vi "Read Attribute Data.vi"(8 "error in (no error)":errorcluster, 10 "Object Name":string, 11 "BNT_BlowfishFactory in":refnum<class "BNT_BlowfishFactory.lvclass">) -> (0 "error out":errorcluster, 2 "Attribute Data":variant, 3 "BNT_BlowfishFactory out":refnum<class "BNT_BlowfishFactory.lvclass">)   [LabVIEW 2018, in "BNT_Factories.lvlib" / "BNT_BlowfishFactory.lvclass"]
doc: "Read object attribute data from storage medium.\n\nThe default implementation reads from ini-file."
uses:
  BNT_BlowfishFactory.lvclass
  C:/User/Brand/LVP/BNT/TempCtrl/Packages/CSPP_Core/Classes/CSPP_BaseClasses/Factory/CSPP_Factory.lvclass
  CSPP_Core/Classes/CSPP_BaseClasses/Factory/CSPP_Factory.lvclass/CSPP_Factory.ctl
  BNT_BlowfishFactory.lvclass/BNT_BlowfishFactory.ctl
  CSPP_Core/Classes/CSPP_BaseClasses/Factory/CSPP_Factory.lvclass
  BlowFish/Source/BlowFish.lvlib
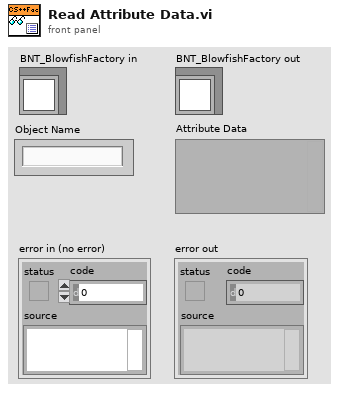
[diagram p1: front panel]
types:
  T1 = enum16{"open", "replace", "create", "open or create", "replace or create", "replace or create with confirmation"}
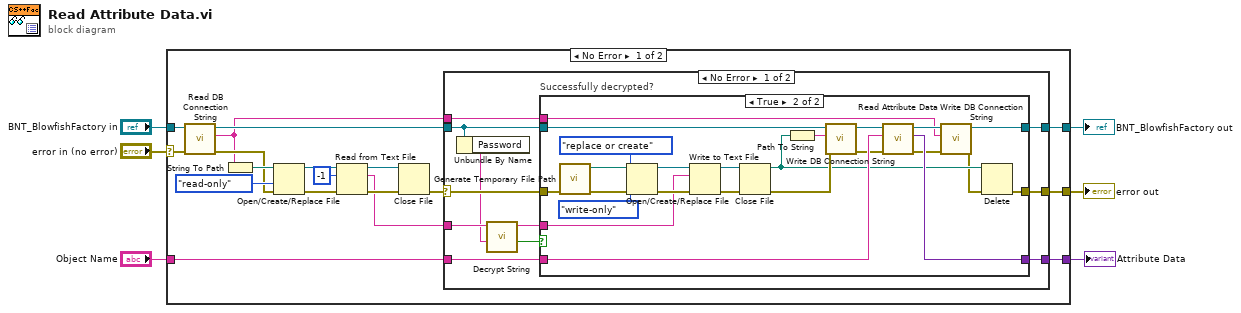
[diagram p0: block diagram]
diagram:
  n1 = case shown="No Error" "error in (no error)" {
    selector: "error in (no error)" -> [w24 w65]
    tunnel: [w9 w65] -> w5
    tunnel: [w11 w64] -> w3
    tunnel: "BNT_BlowfishFactory in" -> [w23 w64]
    tunnel: [w17 _] -> w2
    tunnel: "Object Name" -> [w16 _]
    frame No Error {
      n2 = call "Read DB Connection String.vi"("error in (no error)"=w24, "CS++Factory in"=w23) -> ("error out"=w20:errorcluster, "DB Connection String"=w10:string, "CS++Factory out"=w12:refnum<class "BNT_BlowfishFactory.lvclass">)  [unwired: 7 in]
      n3 = String To Path(string=w10) -> (path=w22:path)
      n4 = Open/Create/Replace File(file path (use dialog)=w22, error in=w20, access (0:read/write)=enum16{"read/write", "read-only", "write-only"}."read-only") -> (refnum out=w19:refnum<file>, error out=w18:errorcluster)  [unwired: 3 in, 1 out]
      n5 = Read from Text File(file (use dialog)=w19, count=-1, error in=w18) -> (refnum out=w14:refnum<file>, text=w7:string, error out=w15:errorcluster)  [unwired: 1 in, 1 out]
      n6 = Close File(refnum=w14, error in=w15) -> (error out=w8:errorcluster)  [unwired: 1 out]
      n7 = case shown="No Error" w8 {
        selector: w8 -> [w30 w62]
        tunnel: [w35 _] -> w17
        tunnel: w16 -> [w34 _]
        tunnel: w12 -> [w27 w63]
        tunnel: [w33 w63] -> w11
        tunnel: w10 -> [w32 _]
        tunnel: [w31 w62] -> w9
        tunnel: w7 -> [w29 _]
        frame No Error {
          n8 = Unbundle By Name(w27) -> ("Password"=w26:string)
          n9 = call "Decrypt String.vi"("Crypto Key"=w26, "Encrypted String"=w29) -> ("Success"=w25:bool, "Decrypted String"=w28:string)  [unwired: 8 in]
          n10 = case "Successfully decrypted?" shown="True" w25 {
            tunnel: [_ w61] -> w35
            tunnel: w34 -> [_ w60]
            tunnel: [w37 w46] -> w33
            tunnel: w32 -> [_ w45]
            tunnel: [w36 w41] -> w31
            tunnel: w30 -> [w36 w40]
            tunnel: w28 -> [_ w39]
            tunnel: w27 -> [w37 w38]
            frame False {
            }
            frame True {
              n11 = call <vilib>:"Generate Temporary File Path.vi"("error in (no error)"=w40) -> ("error out"=w56:errorcluster, "Unique Temporary File Path"=w59:path)  [unwired: 9 in]
              n12 = Open/Create/Replace File(file path (use dialog)=w59, error in=w56, operation (0:open)=T1."replace or create", access (0:read/write)=enum16{"read/write", "read-only", "write-only"}."write-only") -> (refnum out=w55:refnum<file>, error out=w54:errorcluster)  [unwired: 2 in, 1 out]
              n13 = Write to Text File(file (use dialog)=w55, text=w39, error in=w54) -> (refnum out=w52:refnum<file>, error out=w51:errorcluster)  [unwired: 1 in, 1 out]
              n14 = Close File(refnum=w52, error in=w51) -> (path=w44:path, error out=w50:errorcluster)
              n15 = Path To String(path=w44) -> (string=w49:string)
              n16 = call "Write DB Connection String.vi"("error in (no error)"=w50, "DB Connection String"=w49, "CS++Factory in"=w38) -> ("error out"=w48:errorcluster, "CS++Factory out"=w53:refnum<class "BNT_BlowfishFactory.lvclass">)  [unwired: 7 in]
              n17 = call-parent "Read Attribute Data.vi"("error in (no error)"=w48, "Object Name"=w60, "CSPP_Factory in"=w53) -> ("error out"=w43:errorcluster, "Attribute Data"=w61:variant, "CSPP_Factory out"=w47:refnum<class "BNT_BlowfishFactory.lvclass">)  [unwired: 6 in]
              n18 = call "Write DB Connection String.vi"("error in (no error)"=w43, "DB Connection String"=w45, "CS++Factory in"=w47) -> ("error out"=w42:errorcluster, "CS++Factory out"=w46:refnum<class "BNT_BlowfishFactory.lvclass">)  [unwired: 7 in]
              n19 = Delete(path (use dialog)=w44, error in=w42) -> (error out=w41:errorcluster)  [unwired: 3 in, 2 out]
            }
          }
        }
        frame Error {
        }
      }
    }
    frame Error {
    }
  }
  "error out" <- w5
  "BNT_BlowfishFactory out" <- w3
  "Attribute Data" <- w2
